vi "GetGridValue.vi"(8 "error in (no error)":errorcluster, 10 "Coordinate":T2, 11 "SnakeGame in":refnum<class "SnakeGame.lvclass">) -> (0 "error out":errorcluster, 2 "Value":T1 items=["Empty", "Snake1", "Snake2", "Score", "Speed", "Slow"], 3 "SnakeGame out":refnum<class "SnakeGame.lvclass">)   [LabVIEW 2019, in "RT_Game.lvlib" / "SnakeGame.lvclass"]
uses:
  SnakeGame.lvclass
  Game/Coordinate.ctl
  GridValue.ctl
  SnakeGame.lvclass/SnakeGame.ctl
  Game/Game.lvclass
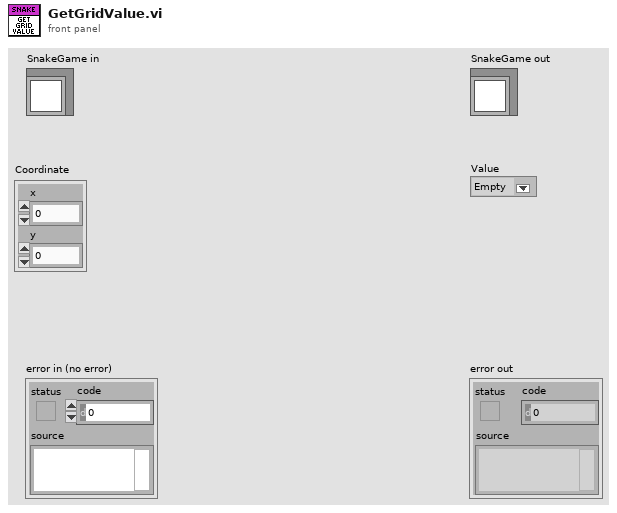
[diagram p1: front panel]
types:
  T1 = typedef "RT_Game.lvlib/SnakeGame.lvclass/GridValue.ctl" = u16
  T2 = typedef "RT_Game.lvlib/Game.lvclass/Coordinate.ctl" = cluster{"x":dbl, "y":dbl}
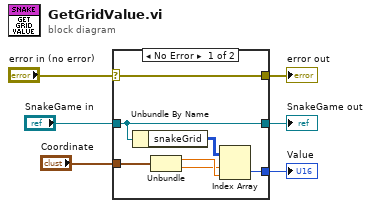
[diagram p0: block diagram]
diagram:
  n1 = case shown="No Error" "error in (no error)" {
    selector: "error in (no error)" -> [w13 w15]
    tunnel: [w13 w15] -> w5
    tunnel: [w12 w14] -> w3
    tunnel: "SnakeGame in" -> [w12 w14]
    tunnel: "Coordinate" -> [w10 _]
    tunnel: [w7 _] -> w1
    frame No Error {
      n2 = Unbundle By Name(w12) -> ("snakeGrid"=w11:u32[][])
      n3 = Unbundle(w10) -> ("x"=w9:dbl, "y"=w8:dbl)
      n4 = Index Array(array=w11, index (row)=w8, index (col)=w9) -> (element=w7:u32)
    }
    frame Error {
    }
  }
  "error out" <- w5
  "SnakeGame out" <- w3
  "Value" <- w1
